vi "Test VI.vi"() -> ()   [LabVIEW 2018]
uses:
  <vilib>/regexp/Match Regular Expression.xnode
panel:
  out "offset past match 2":i32
  out "offset past match":i32
  out "whole match":string
  out "before match":string
  out "after match":string
  out "resulting string":string
  out "Array":string[](array[string])
  out "Array of Strings":string[](array[string])
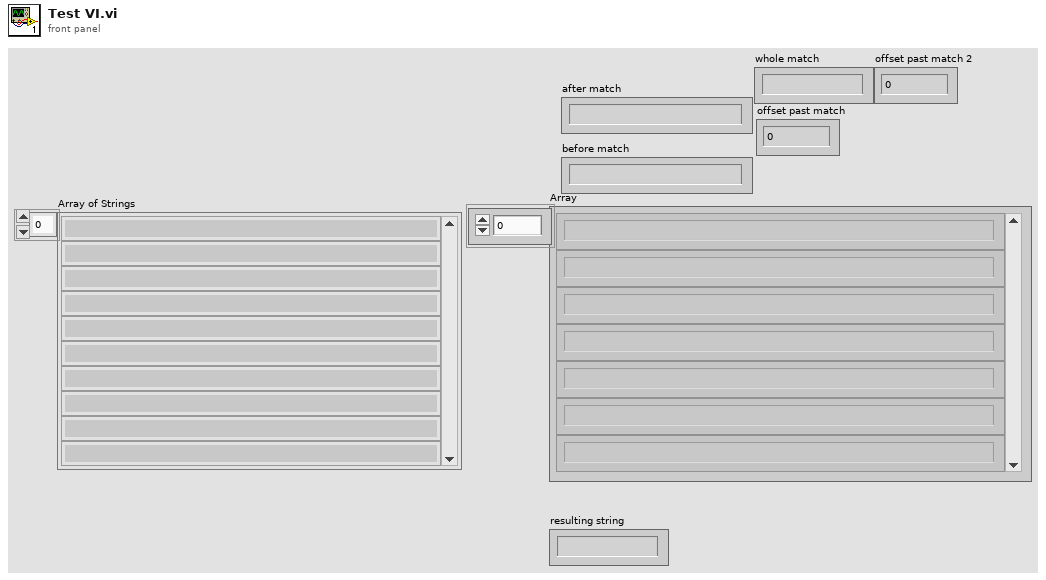
[diagram p1: front panel]
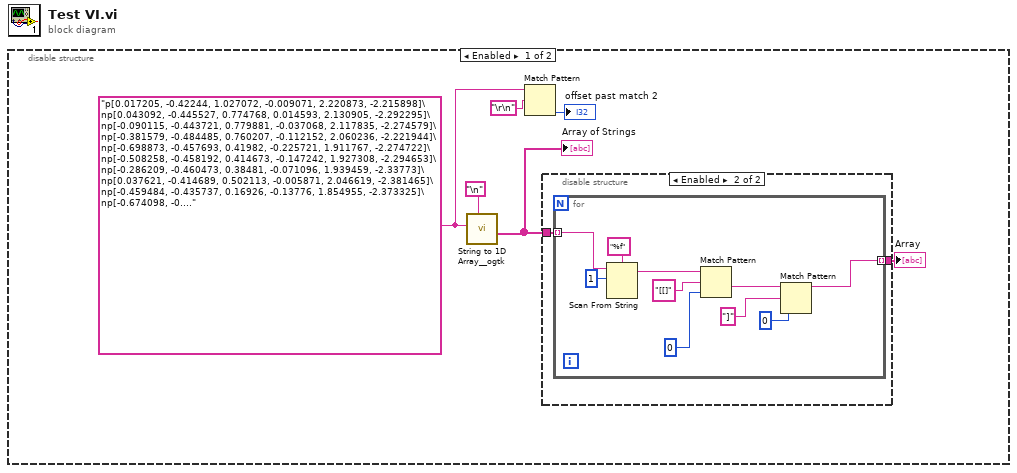
[diagram p0: block diagram]
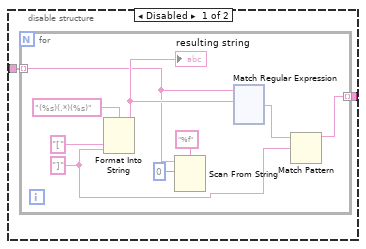
[diagram p2: hidden frame]
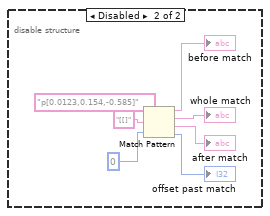
[diagram p3: hidden frame]
diagram:
  n1 = disable-structure shown="Enabled" {
    frame Enabled {
      w3 = "p[0.017205, -0.42244, 1.027072, -0.009071, 2.220873, -2.215898]\np[0.043092, -0.445527, 0.774768, 0.014593, 2.130905, -2.292295]\np[-0.090115, -0.443721, 0.779881, -0.037068, 2.117835, -2.274579]\np[-0.381579, -0.484485, 0.760207, -0.112152, 2.060236, -2.221944]\np[-0.698873, -0.457693, 0.41982, -0.225721, 1.911767, -2.274722]\np[-0.508258, -0.458192, 0.414673, -0.147242, 1.927308, -2.294653]\np[-0.286209, -0.460473, 0.38481, -0.071096, 1.939459, -2.33773]\np[0.037621, -0.414689, 0.502113, -0.005871, 2.046619, -2.381465]\np[-0.459484, -0.435737, 0.16926, -0.13776, 1.854955, -2.373325]\np[-0.674098, -0.478061, 0.183343, -0.204937, 1.829951, -2.332598]\np[0.101275, -0.446982, 0.774179, 0.041979, 2.134068, -2.298833]\np[0.391006, -0.447696, 0.844637, -0.131966, -2.118383, 2.236308]\np[0.693465, -0.450603, 0.411085, -0.203875, -1.921876, 2.308554]\np[0.475784, -0.44847, 0.388518, -0.12633, -1.938008, 2.335226]\np[0.342386, -0.437751, 0.377886, -0.114667, -1.967924, 2.382313]\np[0.452432, -0.433971, 0.13977, -0.127157, -1.869051, 2.418521]\np[0.669213, -0.473436, 0.155507, -0.187034, -1.839432, 2.373627]"
      n2 = call <userlib>:"String to 1D Array__ogtk.vi"("delimiter (Tab)"="\n", "string"=w3) -> ("Array of Strings"=w5:string[])  [unwired: 9 in]
      "Array of Strings" <- w5
      n3 = Match Pattern(string=w3, regular expression="\r\n") -> (offset past match=→"offset past match 2":i32)  [unwired: 1 in, 3 out]
      n4 = disable-structure shown="Enabled" {
        disable-tunnel: w5 -> [w8 w133]
        disable-tunnel: [w7 w132] -> w4
        frame Disabled {
          n5 = for {
            tunnel: w8 -> [w9] mode=indexing
            tunnel: [w10] -> w7 mode=indexing
            w11 = "]"
            n6 = Format Into String(format string="(%s)(.*)(%s)" ("initial string"), "[", w11) -> (resulting string=w15:string)  [unwired: 2 in, 1 out]
            "resulting string" <- w15
            n7 = Scan From String(format string="%f", input string=w9, initial scan location=0) -> ()  [unwired: 3 in, 3 out]
            n8 = xnode "Match Regular Expression"("input string"=w9, "regular expression"=w15) -> ("after match"=w12:string)  [unwired: 4 in, 4 out]
            n9 = Match Pattern(string=w12, regular expression=w11) -> (before substring=w10:string)  [unwired: 1 in, 3 out]
          }
        }
        frame Enabled {
          n10 = for {
            tunnel: w133 -> [w141] mode=indexing
            tunnel: [w134] -> w132 mode=indexing
            n11 = Scan From String(format string="%f", input string=w141, initial scan location=u32 1) -> (remaining string=w140:string)  [unwired: 3 in, 2 out]
            n12 = Match Pattern(string=w140, regular expression="[[]", offset (0)=0) -> (after substring=w136:string)  [unwired: 3 out]
            n13 = Match Pattern(string=w136, regular expression="]", offset (0)=0) -> (before substring=w134:string)  [unwired: 3 out]
          }
        }
      }
      "Array" <- w4
    }
    frame Disabled {
      n14 = Match Pattern(string="p[0.0123,0.154,-0.585]", regular expression="[[]", offset (0)=0) -> (before substring=→"before match":string, match substring=→"whole match":string, after substring=→"after match":string, offset past match=→"offset past match":i32)
    }
  }
